vi "DO Write.vi"(8 "error in (no error)":errorcluster, 10 "Digital Output":bool, 11 "Binary Valve in":refnum<class "Binary Valve.lvclass">) -> (0 "error out":errorcluster)   [LabVIEW 2021, in "Binary Valve.lvlib" / "Binary Valve.lvclass"]
uses:
  Binary Valve.lvclass
  Binary Valve.lvclass/Binary Valve.ctl
  <vilib>/NathanCo/Digital Tasks/Digital Output/Digital Output/Digital Output.lvclass
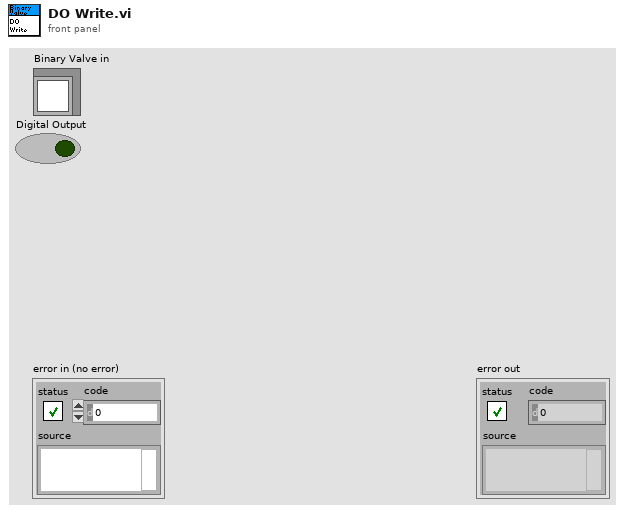
[diagram p1: front panel]
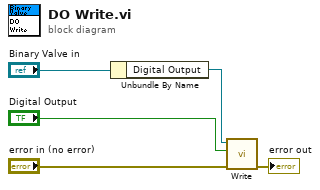
[diagram p0: block diagram]
diagram:
  n1 = Unbundle By Name("Binary Valve in") -> ("Digital Output"=w1:refnum<class "Digital Output.lvclass">)
  n2 = call <vilib>:"Write.vi"("error in (no error)"="error in (no error)", "Digital Output"="Digital Output", "Digital Output in"=w1) -> ("error out"=→"error out":errorcluster)  [unwired: 8 in]
